vi "utility_remove it later.vi"(0 "pulse_gen_and_detect_p2p out":refnum<class "pulse_gen_and_detect_p2p.lvclass">, 11 "error out":errorcluster) -> (4 "pulse_gen_and_detect_p2p out 2":refnum<class "pulse_gen_and_detect_p2p.lvclass">, 15 "error out 2":errorcluster)   [LabVIEW 2021, in "pulse_gen_and_detect_p2p.lvclass"]
uses:
  pulse_gen_and_detect_p2p.lvclass
  pulse_gen_and_detect_p2p.lvclass/pulse_gen_and_detect_p2p.ctl
  <resource>/objmgr/PeerToPeerStream.rc
  <vilib>/userdefined/niP2PState.ctl
panel:
  out "Reader:Underflow":bool
  out "Reader:Size in Elements":u32
  out "Reader:Number of Elements for Reading":u32
  out "Writer:Overflow":bool
  out "Writer:Size in Elements":u32
  out "Writer:Number of Elements for Writing":u32
  out "State":T1
  in  "error in (no error)":errorcluster
  in  "index":i32
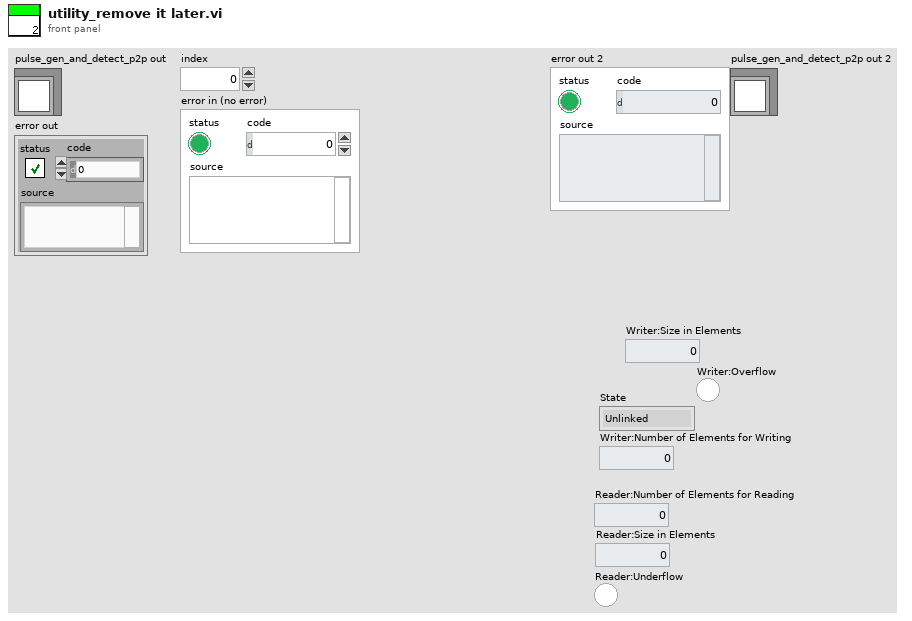
[diagram p1: front panel]
types:
  T1 = typedef "niP2PState.ctl" = enum32{"Unlinked", "Disabled", "Enabled", "Flushing"}
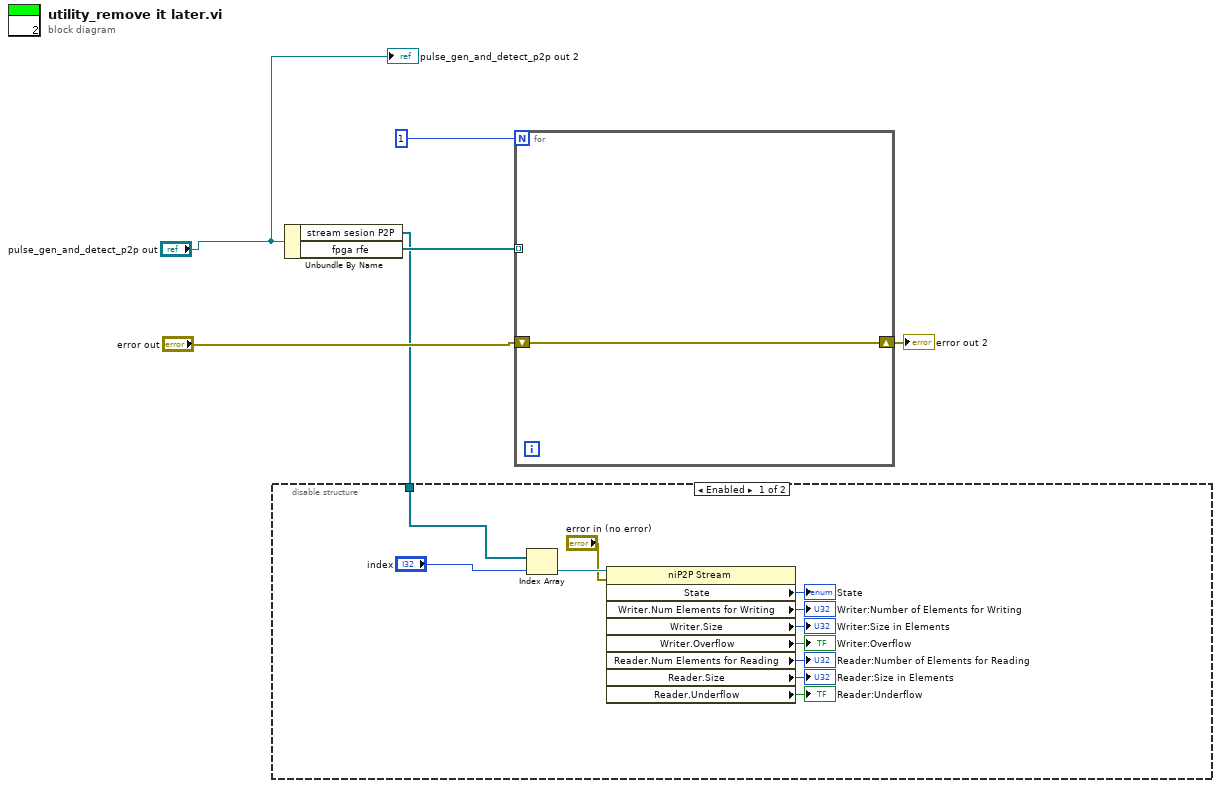
[diagram p0: block diagram]
diagram:
  n1 = Unbundle By Name("pulse_gen_and_detect_p2p out") -> ("stream sesion P2P"=w1:refnum<k20>[], "fpga rfe"=w5:refnum<k20>[])
  n2 = disable-structure shown="Enabled" {
    disable-tunnel: w1 -> [w17 _]
    frame Enabled {
      n3 = Index Array(array=w17, index="index") -> (element=w16:refnum<k20>)
      n4 = property class="niP2P Stream"(reference=w16, error in="error in (no error)") -> ("State"=→"State":T1, "Writer.Num Elements for Writing"=→"Writer:Number of Elements for Writing":u32, "Writer.Size"=→"Writer:Size in Elements":u32, "Writer.Overflow"=→"Writer:Overflow":bool, "Reader.Num Elements for Reading"=→"Reader:Number of Elements for Reading":u32, "Reader.Size"=→"Reader:Size in Elements":u32, "Reader.Underflow"=→"Reader:Underflow":bool)  [unwired: 2 out]
    }
    frame Disabled {
    }
  }
  n5 = for {
    N: 1 -> [_]
    tunnel: w5 -> [_] mode=indexing
    shift-right: [w18] -> w2
    shift-left: "error out" -> [w18]
  }
  "error out 2" <- w2
  "pulse_gen_and_detect_p2p out 2" <- "pulse_gen_and_detect_p2p out"
